vi "Read configuration.vi"(7 "force loading?":bool=TRUE, 8 "error in (no error)":errorcluster, 11 "DAQCascade512 in":refnum<class "DAQCascade512.lvclass">) -> (0 "error out":errorcluster, 3 "DAQCascade512 out":refnum<class "DAQCascade512.lvclass">)   [LabVIEW 2012, in "DAQCascade512.lvclass"]
doc: "Reads the XML-based configuration file and populates the configuration cluster accordingly. Configuration file name is <component ID>.xml."
uses:
  DAQCascade512.lvclass
  <vilib>/Distrio/Murmex/Murmex/Murmex.lvclass
  DAQCascade512.lvclass/DAQCascade512.ctl
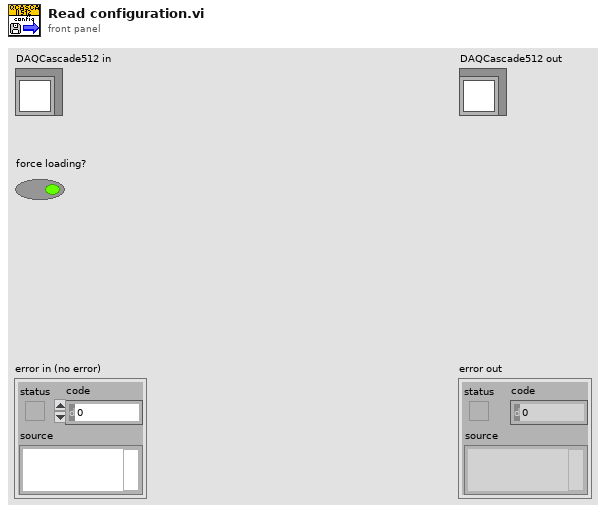
[diagram p1: front panel]
types:
  T1 = typedef "DAQCascade512.lvclass/configuration cluster.ctl" = cluster{"Camera configuration":cluster{"Temperature":dbl, "EMGain":dbl, "ClearMode":T2, "ReadoutMode":T3, "ADC Gain":T4}, "Acqusition Info":cluster{"Image type":T5, "Acquire / Focus Flag":u32}}
  T2 = typedef "Clearing_mode.ctl" = dbl
  T3 = typedef "Readout_mode.ctl" = dbl
  T4 = typedef "ADC_gain.ctl" = i32
  T5 = typedef "Image_type.ctl" = u32
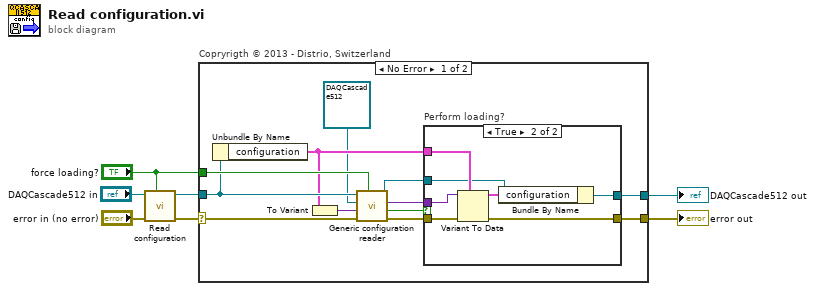
[diagram p0: block diagram]
diagram:
  n1 = call-parent "Read configuration.vi"("force loading?"="force loading?", "error in (no error)"="error in (no error)", "Murmex in"="DAQCascade512 in") -> ("error out"=w2:errorcluster, "Murmex out"=w3:refnum<class "DAQCascade512.lvclass">)  [unwired: 7 in]
  n2 = case "Copryrigth © 2013 - Distrio, Switzerland" shown="No Error" w2 {
    selector: w2 -> [w16 w30]
    tunnel: [w18 w30] -> w4
    tunnel: [w19 w29] -> w5
    tunnel: w3 -> [w13 w29]
    tunnel: "force loading?" -> [w17 _]
    frame No Error {
      n3 = Unbundle By Name(w13) -> ("configuration"=w11:T1)
      n4 = To Variant(anything=w11) -> (Variant=w12:variant)
      n5 = call <vilib>:"Generic configuration reader.vi"("force loading?"=w17, "error in (no error)"=w16, "configuration cluster variant"=w12, "inheritance level"=refnum<class "DAQCascade512.lvclass"> refnum ("DAQCascade512"), "Murmex in"=w13) -> ("error out"=w15:errorcluster, "loaded?"=w9:bool, "configuration data (variant)"=w10:variant, "Murmex out"=w14:refnum<class "DAQCascade512.lvclass">)  [unwired: 3 in]
      n6 = case "Perform loading?" shown="True" w9 {
        tunnel: [w21 w23] -> w19
        tunnel: w11 -> [_ w28]
        tunnel: [w20 w22] -> w18
        tunnel: w15 -> [w20 w25]
        tunnel: w14 -> [w21 w27]
        tunnel: w10 -> [_ w24]
        frame False {
        }
        frame True {
          n7 = Variant To Data(error in=w25, type=w28, Variant=w24) -> (data=w26:T1, error out=w22:errorcluster)
          n8 = Bundle By Name(cluster=w27, "configuration"=w26) -> (w23:refnum<class "DAQCascade512.lvclass">)
        }
      }
    }
    frame Error {
    }
  }
  "error out" <- w4
  "DAQCascade512 out" <- w5
